vi "engine.vi"   [LabVIEW 2020, in "eos.lvlib" / "statemachine.lvclass"]
uses:
  statemachine.lvclass
  interfaces/state/state.lvclass
  states/shutting-down/shuttingDown.lvclass
  C:/Projects/LVOS/EngineeringOS/source/classes/states/shutting-down/shuttingDown.lvclass
  C:/Projects/LVOS/EngineeringOS/source/interfaces/state/state.lvclass
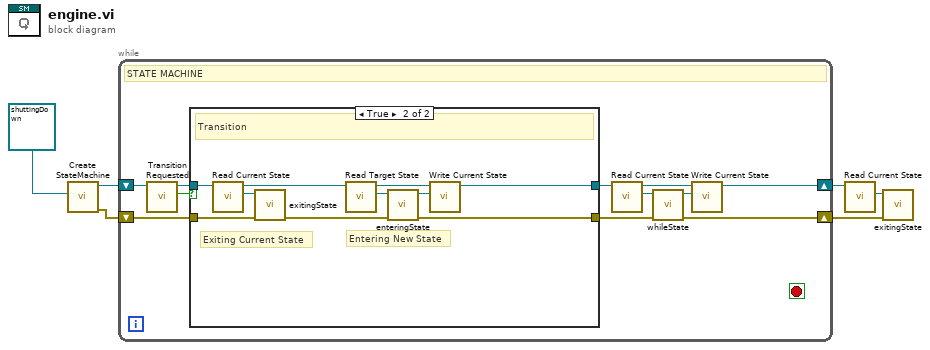
[diagram p0: block diagram]
diagram:
  n1 = call "Create StateMachine.vi"("Final State"=refnum<class "shuttingDown.lvclass"> refnum ("eos.lvlib:shuttingDown.lvclass")) -> ("error out"=w3:errorcluster, "statemachine out"=w4:refnum<class "statemachine.lvclass">)  [unwired: 9 in]
  n2 = while {
    shift-right: [w11] -> w6
    shift-left: w3 -> [w17]
    shift-right: [w12] -> w2
    shift-left: w4 -> [w16]
    stop <- _ stop-if-true
    # "STATE MACHINE"
    n3 = call "Transition Requested.vi"("statemachine"=w16) -> ("Transition Requested?"=w14:bool, "statemachine"=w15:refnum<class "statemachine.lvclass">)  [unwired: 9 in]
    n4 = case shown="True" w14 {
      tunnel: w15 -> [w19 w27]
      tunnel: w17 -> [w18 w28]
      tunnel: [w18 w20] -> w10
      tunnel: [w19 w23] -> w13
      frame False {
        # "No Transition"
      }
      frame True {
        # "Entering New State"
        # "Exiting Current State"
        # "Transition"
        n5 = call "Read Current State.vi"("statemachine in"=w27) -> ("Current State"=w29:refnum<class "state.lvclass">, "statemachine out"=w22:refnum<class "statemachine.lvclass">)  [unwired: 9 in]
        n6 = call-dynamic "exitingState.vi"("error in (no error)"=w28, "state in"=w29) -> ("error out"=w21:errorcluster)  [unwired: 8 in, 1 out]
        n7 = call "Read Target State.vi"("statemachine in"=w22) -> ("Target State"=w25:refnum<class "state.lvclass">, "statemachine out"=w26:refnum<class "statemachine.lvclass">)  [unwired: 9 in]
        n8 = call-dynamic "enteringState.vi"("error in (no error)"=w21, "state in"=w25) -> ("error out"=w20:errorcluster, "state out"=w24:refnum<class "state.lvclass">)  [unwired: 8 in]
        n9 = call "Write Current State.vi"("Current State"=w24, "statemachine in"=w26) -> ("statemachine out"=w23:refnum<class "statemachine.lvclass">)  [unwired: 9 in]
      }
    }
    n10 = call "Read Current State.vi"("statemachine in"=w13) -> ("Current State"=w8:refnum<class "state.lvclass">, "statemachine out"=w9:refnum<class "statemachine.lvclass">)  [unwired: 9 in]
    n11 = call-dynamic "whileState.vi"("error in (no error)"=w10, "state in"=w8) -> ("error out"=w11:errorcluster, "state out"=w7:refnum<class "state.lvclass">)  [unwired: 6 in, 2 out]
    n12 = call "Write Current State.vi"("Current State"=w7, "statemachine in"=w9) -> ("statemachine out"=w12:refnum<class "statemachine.lvclass">)  [unwired: 9 in]
  }
  n13 = call "Read Current State.vi"("statemachine in"=w2) -> ("Current State"=w1:refnum<class "state.lvclass">)  [unwired: 9 in, 1 out]
  n14 = call-dynamic "exitingState.vi"("error in (no error)"=w6, "state in"=w1) -> ()  [unwired: 8 in, 2 out]
